vi "Write Controls refs.vi"(8 "error in (no error)":errorcluster, 10 "Controls refs":T1, 11 "Detector in":refnum<class "Detector.lvclass">) -> (0 "error out":errorcluster, 3 "Detector out":refnum<class "Detector.lvclass">)   [LabVIEW 2015, in "Detector.lvclass"]
uses:
  Detector.lvclass
  Controls-refs_CLIENT.ctl
  Detector.lvclass/Detector.ctl
  Control/Control-Client/Control-Client.lvclass
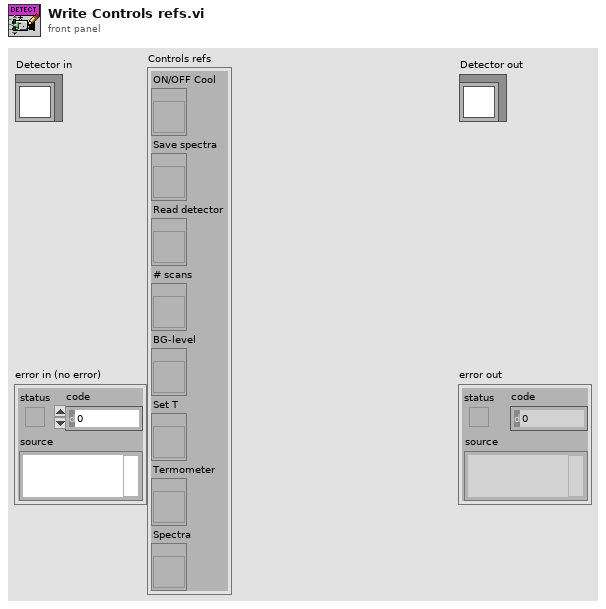
[diagram p1: front panel]
types:
  T1 = typedef "Control-Client.lvclass/Controls-refs_CLIENT.ctl" = cluster{"ON/OFF Cool":refnum<vi>, "Save spectra":refnum<vi>, "Read detector":refnum<vi>, "# scans":refnum<vi>, "BG-level":refnum<vi>, "Set T":refnum<vi>, "Termometer":refnum<vi>, "Spectra":refnum<vi>}
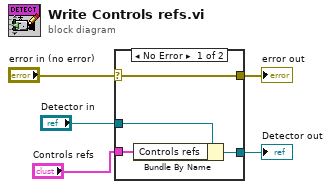
[diagram p0: block diagram]
diagram:
  n1 = case shown="No Error" "error in (no error)" {
    selector: "error in (no error)" -> [w9 w10]
    tunnel: [w9 w10] -> w4
    tunnel: [w7 w11] -> w2
    tunnel: "Detector in" -> [w8 w11]
    tunnel: "Controls refs" -> [w6 _]
    frame No Error {
      n2 = Bundle By Name(cluster=w8, "Controls refs"=w6) -> (w7:refnum<class "Detector.lvclass">)
    }
    frame Error {
    }
  }
  "error out" <- w4
  "Detector out" <- w2
